vi "JKISM++ TopMain.vi"() -> ()   [LabVIEW 2014]
uses:
  user.lib/_NEVSTOP/JKI State Machine ++/_Support/JKISMQ/_JKISMQFGV.vi
  user.lib/_NEVSTOP/JKI State Machine ++/JKI-State-Machine-Plus.lvlib
panel:
  in  "List Module":bool
  out "Name":string[](array[string])
  in  "New Category: 3 -@A":bool
  in  "New Category: 3 ->A":bool
  in  "New Category: 2 -@B":bool
  out "State History":string
  in  "New Category: 2 ->B":bool
  in  "Boolean 1":bool
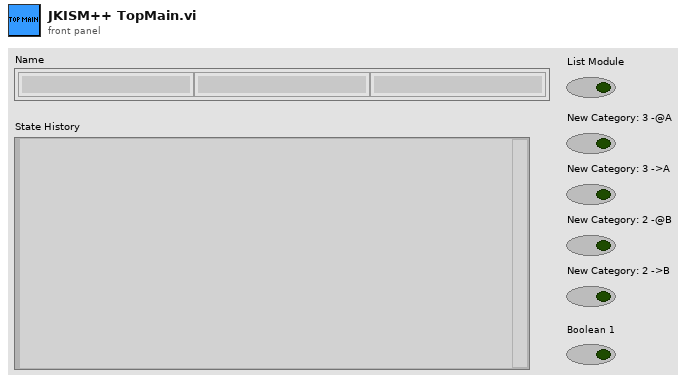
[diagram p1: front panel]
types:
  T1 = enum32{"Invalid", "Standard", "Closed", "Hidden", "Minimized", "Maximized"}
  T2 = enum32{"invalid app kind", "Development System", "Run Time System", "Student Edition", "Embedded LabVIEW", "Evaluation", "Custom"}
  T3 = cluster{"Core":cluster{"Current VI Reference":refnum<vi>, "Close Panel on Exit?":bool}, "Your Boolean data":bool, "Your string data":string}
  T4 = cluster{"Current VI Reference":refnum<vi>, "Close Panel on Exit?":bool}
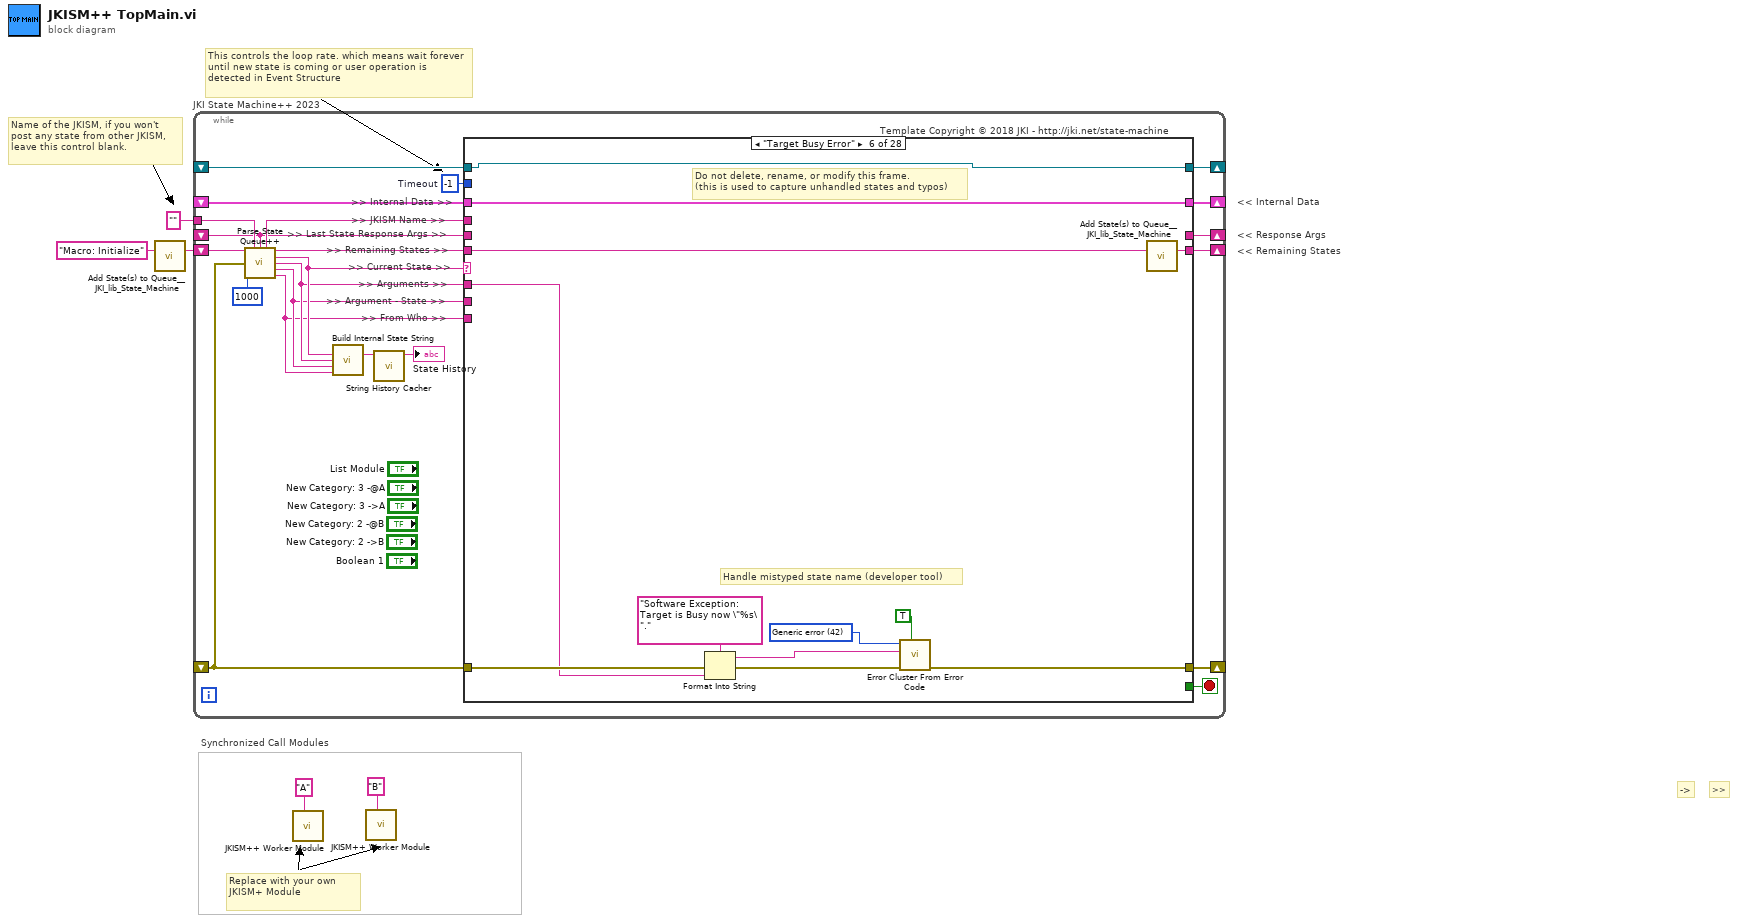
[diagram p0: block diagram]
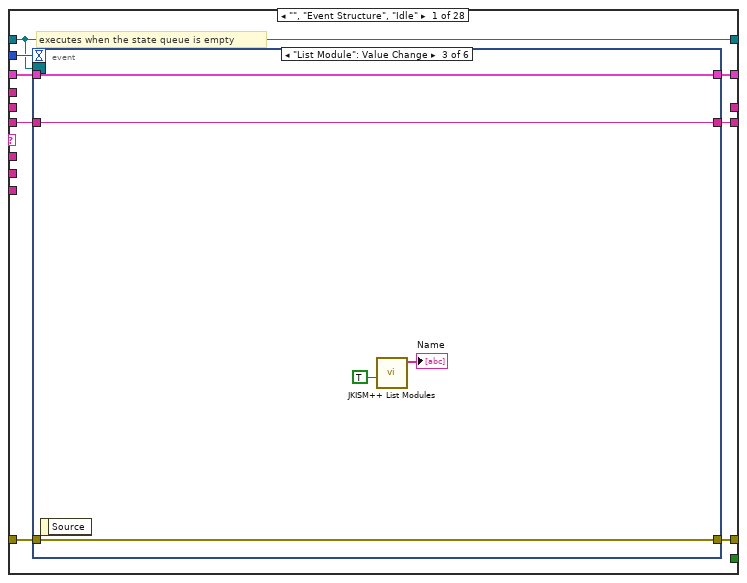
[diagram p2: hidden frame]
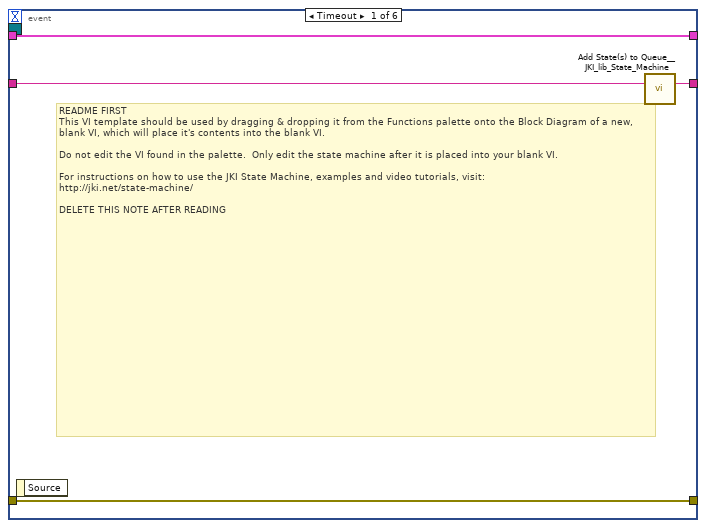
[diagram p3: hidden frame]
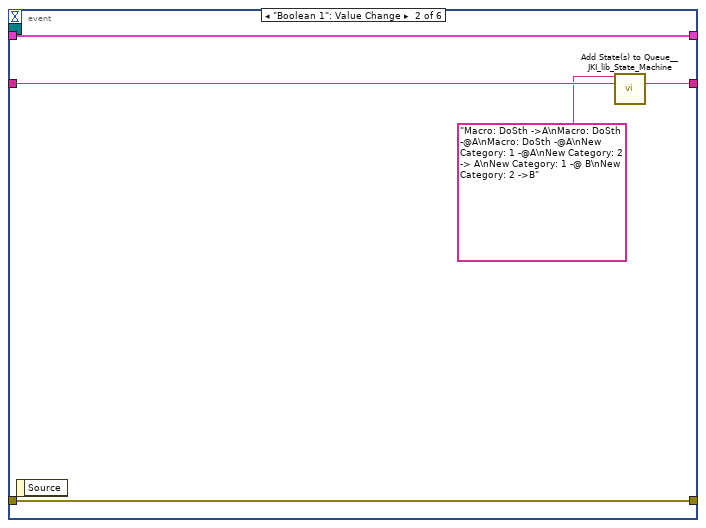
[diagram p4: hidden frame]
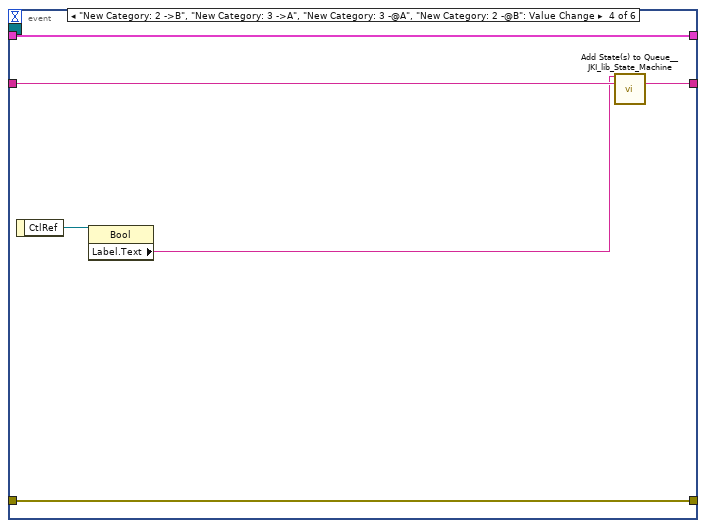
[diagram p5: hidden frame]
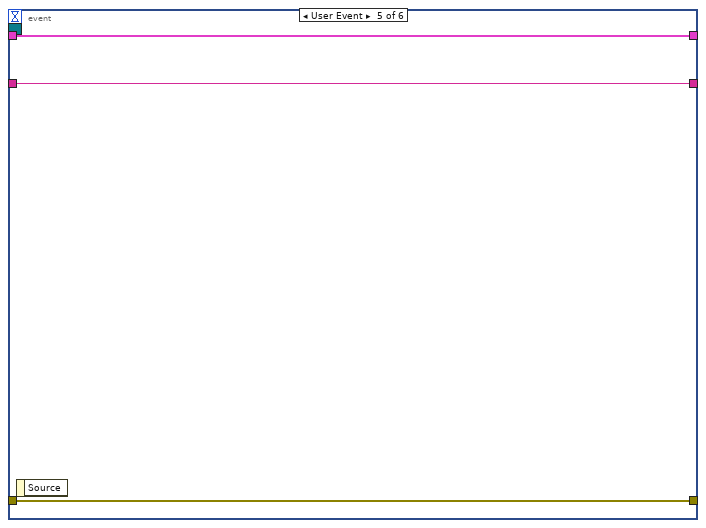
[diagram p6: hidden frame]
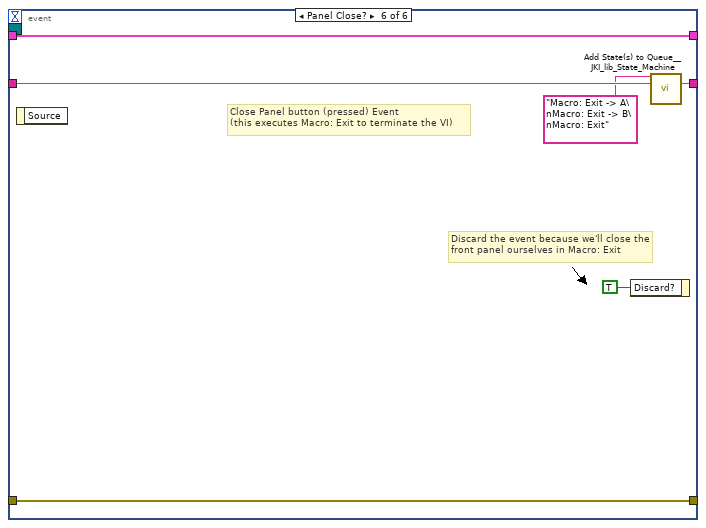
[diagram p7: hidden frame]
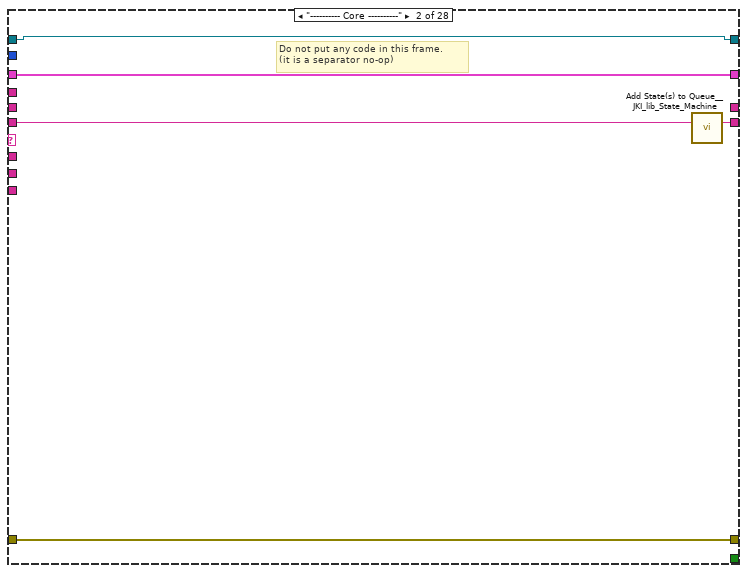
[diagram p8: hidden frame]
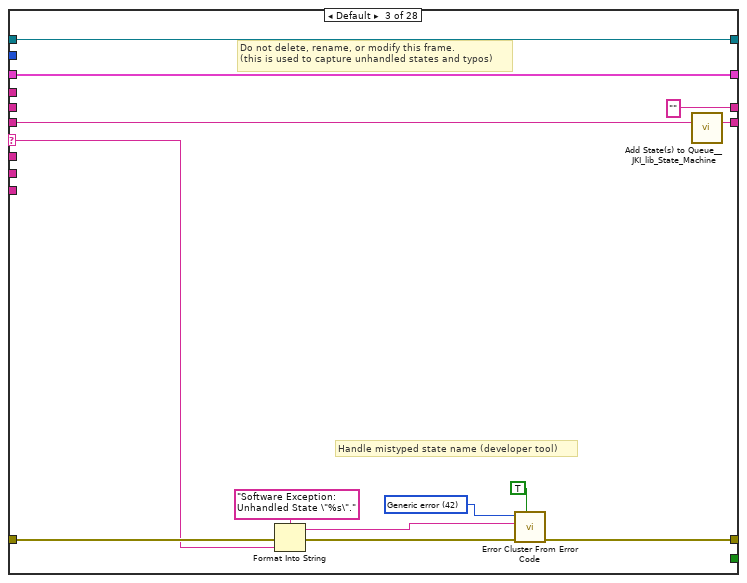
[diagram p9: hidden frame]
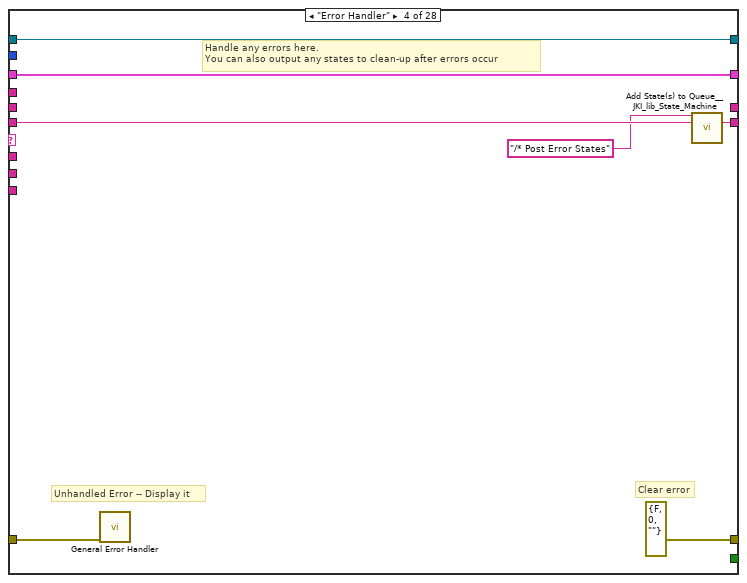
[diagram p10: hidden frame]
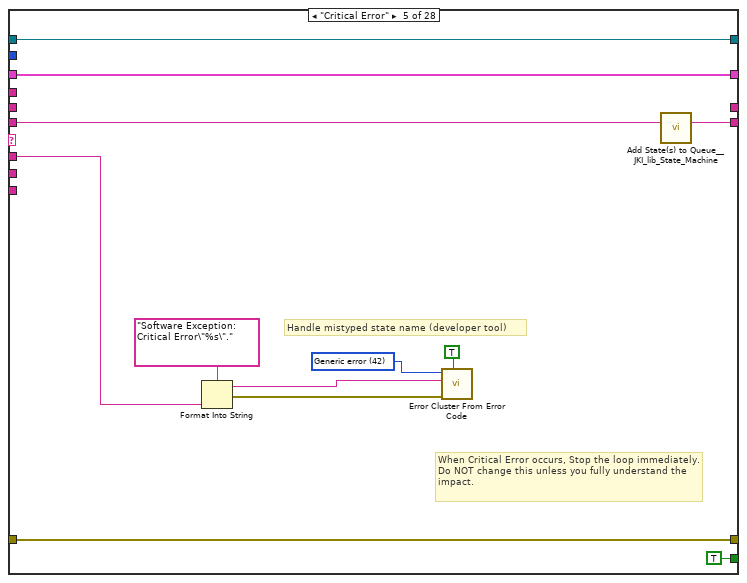
[diagram p11: hidden frame]
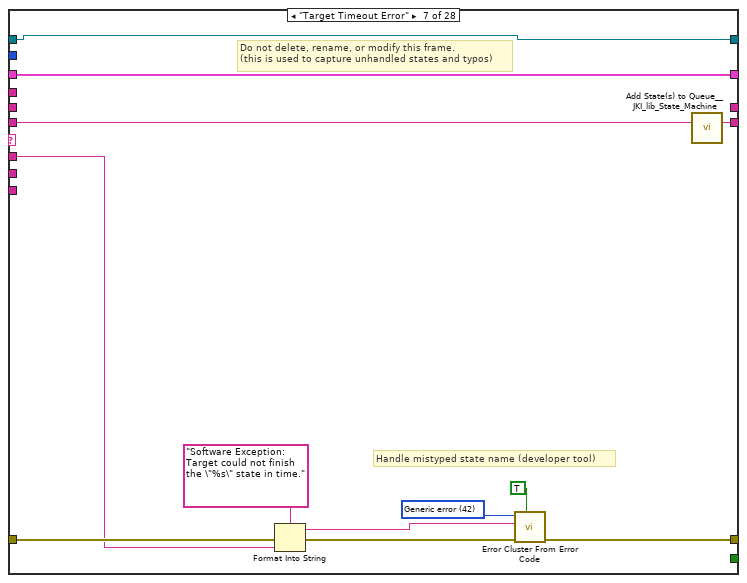
[diagram p12: hidden frame]
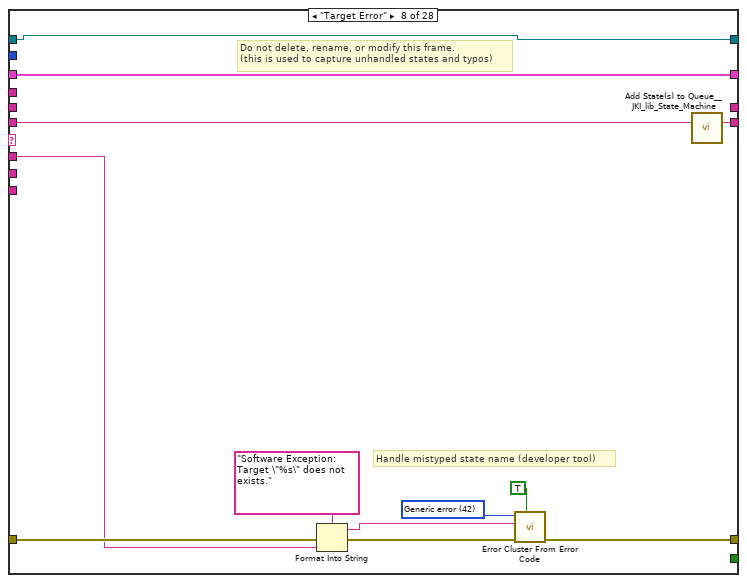
[diagram p13: hidden frame]
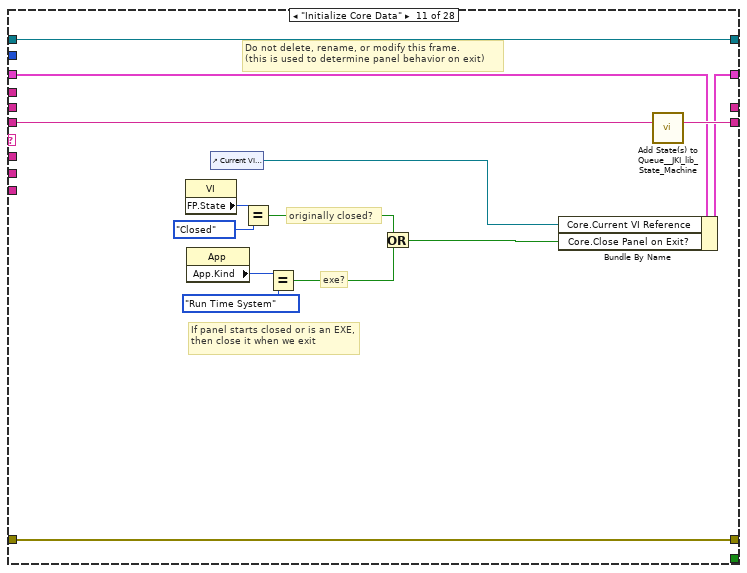
[diagram p16: hidden frame]
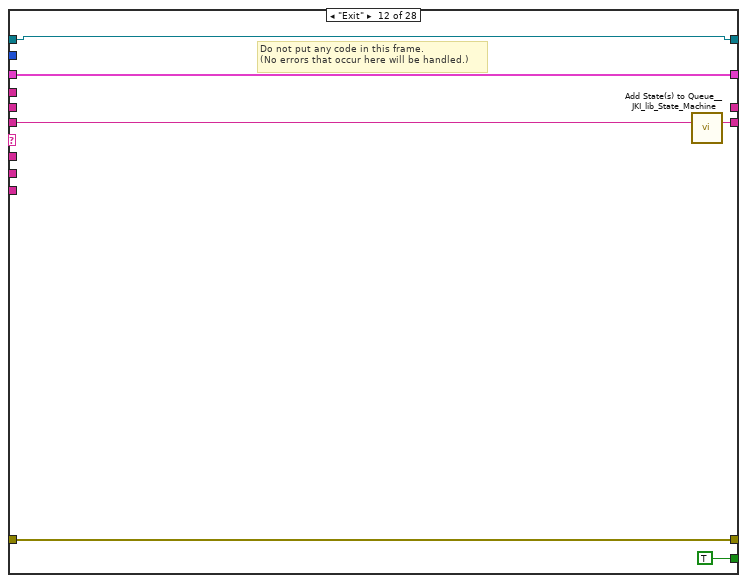
[diagram p17: hidden frame]
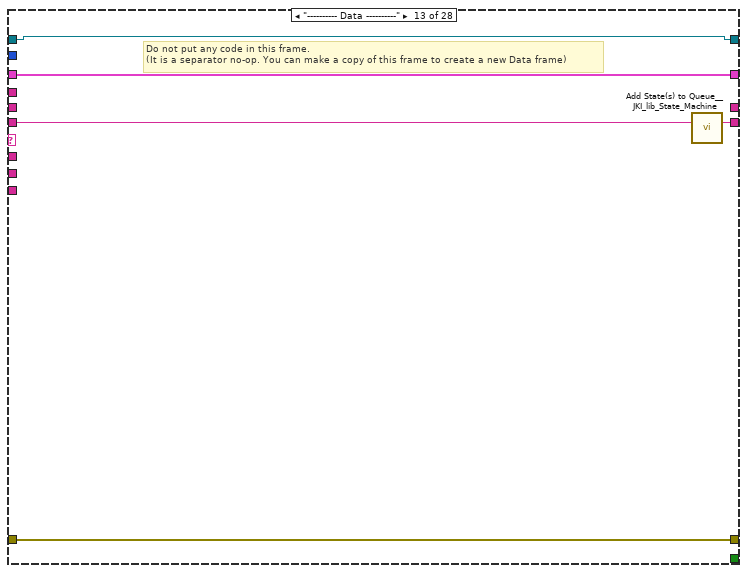
[diagram p18: hidden frame]
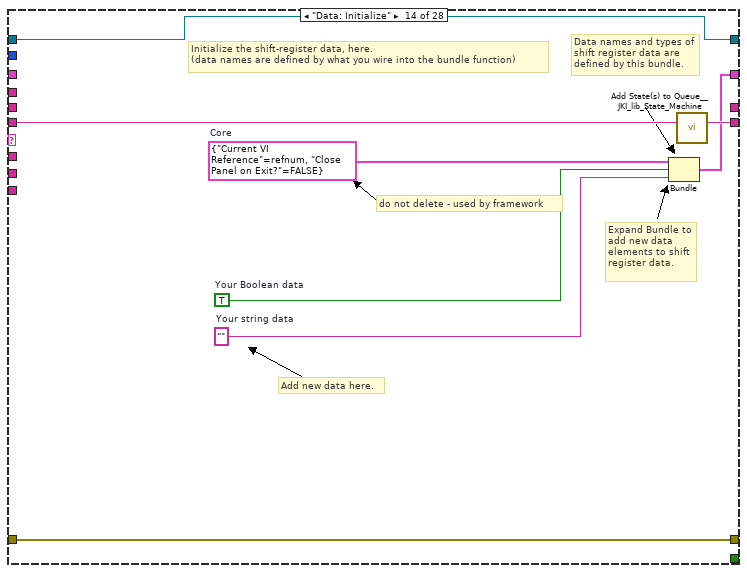
[diagram p19: hidden frame]
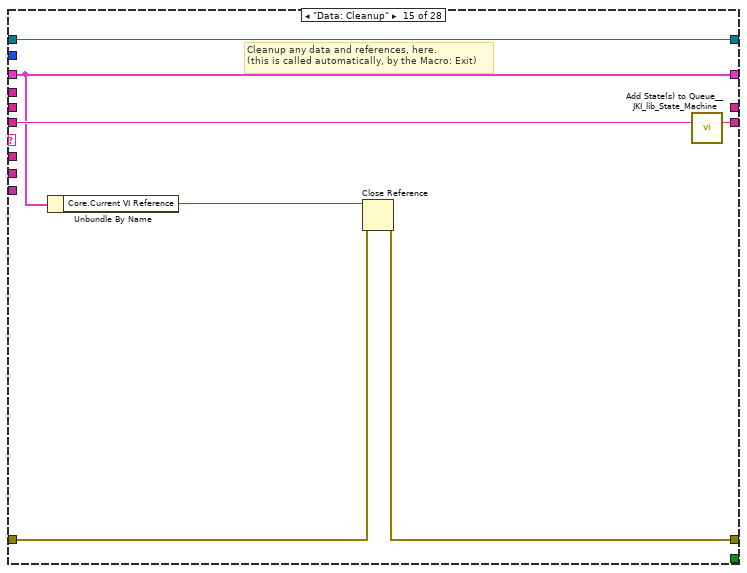
[diagram p20: hidden frame]
diagram:
  # ">>"
  # "->"
  # "<< Internal Data"
  # "<< Response Args"
  # "<< Remaining States"
  # "Name of the JKISM, if you won't post any state from other JKISM,  leave this control blank."
  # "This controls the loop rate. which means wait forever until new state is coming or user operation is detected in Event Structure"
  # "Synchronized Call Modules"
  # "Replace with your own JKISM+ Module"
  n1 = call <vilib>:"Add State(s) to Queue__JKI_lib_State_Machine.vi"("State(s) in (\"\")"="Macro: Initialize") -> ("States Out"=w3:string)  [unwired: 14 in]
  n2 = while "JKI State Machine++ 2023" {
    shift-right: [w22] -> _
    shift-left: _ -> [w21]
    shift-right: [w25] -> _
    shift-left: _ -> [w19]
    shift-right: [w24] -> _
    shift-left: w3 -> [w26]
    tunnel: "" ("Name(\"\" to use uuid)") -> [w14]
    shift-right: [w17] -> _
    shift-left: _ -> [w6]
    shift-right: [w16] -> _
    shift-left: _ -> [w15]
    stop <- w23 stop-if-true
    w20 = -1  # Timeout
    # ">> Internal Data >>"
    # ">> Last State Response Args >>"
    # ">> JKISM Name >>"
    # ">> From Who >>"
    # ">> Argument - State >>"
    # ">> Arguments >>"
    # ">> Current State >>"
    # ">> Remaining States >>"
    # "Template Copyright © 2018 JKI - http://jki.net/state-machine"
    n3 = call "Parse State Queue++.vi"("State Queue"=w26, "Name(\"\" to use uuid)"=w14, "Response Arguments"=w6, "Error In (no error)"=w19, "Response Timeout(5000ms)"=1000 ("Response Timeout(1000ms)")) -> ("Name Used"=w7:string, "Remaining States"=w27:string, "Current State"=w11:string, "Arguments"=w10:string, "Argument - State"=w9:string, "From Who"=w8:string)  [unwired: 5 in]
    n4 = call "Build Internal State String.vi"("State"=w11, "Arguments (\"\")"=w10, "Arg-State (\"\")"=w9, "Source (\"\")"=w8) -> ("State with Arguments"=w12:string)  [unwired: 11 in]
    n5 = call "String History Cacher.vi"("String"=w12) -> ("String Cache"=→"State History":string)  [unwired: 10 in]
    n6 = case shown="\"Target Busy Error\"" w11 {
      selector: w11 -> [_ _ w72 _ _ _ _ _ _ _ _ _ _ _ _ _ _ _ _ _ _ _ _ _ _ _ _ _]
      tunnel: w27 -> [w35 w69 w76 w89 w99 w107 w119 w131 w140 w144 w159 w165 w170 w178 w185 w190 w196 w200 w206 w211 w218 w230 w300 w306 w317 w322 w328 w334]
      tunnel: w10 -> [_ _ _ _ w92 w103 w115 w127 _ _ _ _ _ _ _ _ _ _ _ _ w213 w224 _ _ _ _ _ _]
      tunnel: w21 -> [w33 w66 w74 w86 w100 w105 w117 w129 w139 w143 w152 w163 w167 _ w180 w187 w195 w199 w203 w209 w216 w226 w297 w303 w314 w319 w325 w331]
      tunnel: [w32 w67 w78 errorcluster {"status"=FALSE, "code"=0, "source"=""} ("error out") w101 w109 w121 w133 w141 w145 w156 w162 w168 w175 w181 w188 w191 w198 w204 w208 w214 w227 w298 w304 w315 w320 w326 w332] -> w25
      tunnel: w19 -> [w31 w67 w77 w85 w101 w108 w120 w132 w141 w145 w156 w162 w168 w175 w182 w188 _ w201 w204 w208 w215 w228 w298 w304 w315 w320 w326 w332]
      tunnel: [w34 w68 w75 w88 w98 w106 w118 w130 w140 w144 w158 w164 w169 w177 w184 w189 w196 w200 w205 w210 w217 w229 w299 w305 w316 w321 w327 w333] -> w24
      tunnel: [_ _ _ _ TRUE _ _ _ _ _ _ TRUE _ _ _ _ _ _ _ _ _ _ _ _ _ _ _ _] -> w23
      tunnel: [w30 w66 w74 w86 w100 w105 w117 w129 w139 w143 w157 w163 w167 w176 w180 w187 w195 w199 w203 w209 w216 w226 w297 w303 w314 w319 w325 w331] -> w22
      tunnel: w20 -> [w29 _ _ _ _ _ _ _ _ _ _ _ _ _ _ _ _ _ _ _ _ _ _ _ _ _ _ _]
      tunnel: w8 -> [_ _ _ _ _ _ _ _ _ _ _ _ _ _ _ _ _ _ _ _ _ _ _ _ _ _ _ _]
      tunnel: w9 -> [_ _ _ _ _ _ _ _ _ _ _ _ _ _ _ _ _ _ _ _ _ _ _ _ _ _ _ _]
      tunnel: [_ _ "" _ _ _ _ _ _ _ _ _ _ _ _ _ _ _ _ _ _ _ _ _ _ _ "DoA Finished" "DoB Finished"] -> w17
      tunnel: [w28 w65 w70 w83 w90 w102 w114 w126 w138 w142 w146 w160 w166 w171 w179 w186 w194 w197 w202 w207 w212 w223 w296 w301 w307 w318 w324 w330] -> w16
      tunnel: w15 -> [w28 w65 w70 w83 w90 w102 w114 w126 w138 w142 w146 w160 w166 w171 w179 w186 _ w197 w202 w207 w212 w223 w296 w301 w307 w318 w324 w330]
      tunnel: w7 -> [_ _ _ _ _ _ _ _ _ _ _ _ _ _ _ _ w193 _ _ _ _ _ _ _ _ _ _ _]
      tunnel: w6 -> [_ _ _ _ _ _ _ _ _ _ _ _ _ _ _ _ _ _ _ _ _ _ _ _ _ _ _ _]
      frame "", "Event Structure", "Idle" {
        # "executes when the state queue is empty"
        n7 = event shown="[2] \"List Module\": Value Change" {
          selector: w28 -> [_ _ _ _ _ _]
          dyn-events: _ -> [_ _ _ _ _ _]
          timeout: w29 -> [_ _ _ _ _ _]
          tunnel: w35 -> [w39 w42 w49 w53 w57 w64]
          tunnel: [w38 w41 w49 w52 w57 w63] -> w34
          tunnel: w33 -> [w36 w43 w47 w54 w58 w61]
          tunnel: [w37 w44 w48 w55 w56 w62] -> w32
          tunnel: w31 -> [w37 w44 w48 w55 w56 w62]
          tunnel: [w36 w43 w47 w54 w58 w61] -> w30
          event Timeout {
            # "README FIRST\nThis VI template should be used by dragging & dropping it from the Functions palette onto the Block Diagram of a new, blank VI, which will place it's contents into the blank VI.\n\nDo not edit the VI found in the palette.  Only edit the state machine after it is placed into your blank VI.\n\nFor instructions on how to use the JKI State Machine, examples and video tutorials, visit:\nhttp://jki.net/state-machine/\n\nDELETE THIS NOTE AFTER READING"
            n8 = event-data() -> ()  [unwired: 1 in, 1 out]
            n9 = call <vilib>:"Add State(s) to Queue__JKI_lib_State_Machine.vi"("State(s) in (\"\")"=w39) -> ("States Out"=w38:string)  [unwired: 14 in]
          }
          event "Boolean 1": Value Change {
            n10 = event-data() -> ()  [unwired: 1 in, 1 out]
            n11 = call <vilib>:"Add State(s) to Queue__JKI_lib_State_Machine.vi"("State(s) in Front (\"\")"="Macro: DoSth ->A\nMacro: DoSth -@A\nMacro: DoSth -@A\nNew Category: 1 -@A\nNew Category: 2 -> A\nNew Category: 1 -@ B\nNew Category: 2 ->B" ("State(s) in Front (\"\")"), "State(s) in (\"\")"=w42) -> ("States Out"=w41:string)  [unwired: 13 in]
          }
          event "List Module": Value Change {
            n12 = event-data() -> ()  [unwired: 1 in, 1 out]
            n13 = call "JKISM++ List Modules.vi"("Exclude Standalone JKISM(T)"=TRUE) -> ("Name"=→"Name":string[])  [unwired: 9 in, 1 out]
          }
          event "New Category: 2 ->B", "New Category: 3 ->A", "New Category: 3 -@A", "New Category: 2 -@B": Value Change {
            n14 = event-data() -> ("CtlRef"=w51:refnum<vi>)  [unwired: 1 in]
            n15 = property class="Bool"(reference=w51) -> ("Label.Text"=w50:string)  [unwired: 1 in, 2 out]
            n16 = call <vilib>:"Add State(s) to Queue__JKI_lib_State_Machine.vi"("State(s) in Front (\"\")"=w50, "State(s) in (\"\")"=w53) -> ("States Out"=w52:string)  [unwired: 13 in]
          }
          event User Event {
            n17 = event-data() -> ()  [unwired: 1 in, 1 out]
          }
          event Panel Close? {
            # "Discard the event because we'll close the front panel ourselves in Macro: Exit"
            # "Close Panel button (pressed) Event\n(this executes Macro: Exit to terminate the VI)"
            n18 = event-data() -> ()  [unwired: 1 in, 1 out]
            n19 = event-data("Discard?"=TRUE) -> ()  [unwired: 1 in, 1 out]
            n20 = call <vilib>:"Add State(s) to Queue__JKI_lib_State_Machine.vi"("State(s) in Front (\"\")"="Macro: Exit -> A\nMacro: Exit -> B\nMacro: Exit", "State(s) in (\"\")"=w64) -> ("States Out"=w63:string)  [unwired: 13 in]
          }
        }
      }
      frame "---------- Core ----------" {
        # "Do not put any code in this frame.\n(it is a separator no-op)"
        n21 = call <vilib>:"Add State(s) to Queue__JKI_lib_State_Machine.vi"("State(s) in (\"\")"=w69) -> ("States Out"=w68:string)  [unwired: 14 in]
      }
      frame Default {
        w81 = 42 items=["No error", "Argument error", "Memory is full", "Out of zone", "End of file", "File already open", "Generic file I/O error", "File not found", "File permission error", "Disk is full", "Duplicate path", "Too many files open", "System feature not enabled", "Resource file not found", "Cannot add resource", "Resource not found", "Image not found", "Image memory error", "Pen does not exist", "Config type invalid", "Config token not found", "Config parse error", "Config memory error", "Bad external code format", "Bad external code offset", "External code not present", "Null window", "Destroy window error", "Null menu", "Print aborted", "Bad print record", "Print driver error", "Windows error during printing", "Memory error during printing", "Print dialog error", "Generic print error", "Invalid device refnum", "Device not found", "Device parameter error", "Device unit error", "Cannot open device", "Device call aborted", "Generic error", "Cancelled by user", "Object ID too low", "Object ID too high", "Object not in heap", "Unknown heap", "Unknown object (invalid DefProc)", "Unknown object (DefProc not in table)", "Message out of range", "Invalid (null) method", "Unknown message", "Manager call not supported", "Bad address", "Network operation in progress", "Network operation timed out", "Connection is busy", "Network attribute not supported", "Network error", "Address in use", "System out of memory", "Connection aborted", "Connection refused", "Not connected", "Already connected", "Connection closed", "Initialization error (interapplication manager)", "Bad occurrence", "Wait on unbound occurrence handler", "Occurrence queue overflow", "Datalog type conflict", "Unused", "Unrecognized type (interapplication manager)", "Memory corrupt", "Failed to make temporary DLL", "Old CIN version", "Drag socket not found", "Failed to load drop-object", "Failed to register OLE object", "Failed to release OLE object", "Format specifier type mismatch", "Unknown format specifier", "Too few format specifiers", "Too many format specifiers", "Scan failed", "Newer CIN version", "Error converting to variant", "Runtime menu error", "Password tampered", "Variant attribute not found", "Incompatible variant data type", "Event data is not available", "Event Store is not present", "Occurrence is not found", "Event Queue is not created", "Event info is not available", "Refnum passed is NULL", "Error retrieving Class GUID", "Error retrieving CoClass GUID", "Error retrieving TypeLib GUID.", "Bad built application magic bytes.", "Specific driver is different from the specific driver associated with the Logical Name.", "There is no session opened to the class driver.", "Max Error", "MAX - Error with config objects", "MAX - Error loading configuration", "MAX - Group not supported"]
        # "Do not delete, rename, or modify this frame.\n(this is used to capture unhandled states and typos)"
        # "Handle mistyped state name (developer tool)"
        n22 = Format Into String(format string="Software Exception: Unhandled State \"%s\"." ("message"), error in=w77, w72) -> (resulting string=w80:string, error out=w79:errorcluster)  [unwired: 1 in]
        n23 = call <vilib>:"Error Cluster From Error Code.vi"("show call chain? (False)"=TRUE, "error in (no error)"=w79, "error message (\"\")"=w80, "error code (0)"=w81) -> ("error out"=w78:errorcluster)  [unwired: 5 in]
        n24 = call <vilib>:"Add State(s) to Queue__JKI_lib_State_Machine.vi"("State(s) in (\"\")"=w76) -> ("States Out"=w75:string)  [unwired: 14 in]
      }
      frame "Error Handler" {
        # "Unhandled Error -- Display it"
        # "Handle any errors here.\nYou can also output any states to clean-up after errors occur"
        # "Clear error"
        n25 = call <vilib>:"General Error Handler.vi"("error in (no error)"=w85) -> ()  [unwired: 10 in, 5 out]
        n26 = call <vilib>:"Add State(s) to Queue__JKI_lib_State_Machine.vi"("State(s) in Front (\"\")"="/* Post Error States", "State(s) in (\"\")"=w89) -> ("States Out"=w88:string)  [unwired: 13 in]
      }
      frame "Critical Error" {
        w96 = 42 items=["No error", "Argument error", "Memory is full", "Out of zone", "End of file", "File already open", "Generic file I/O error", "File not found", "File permission error", "Disk is full", "Duplicate path", "Too many files open", "System feature not enabled", "Resource file not found", "Cannot add resource", "Resource not found", "Image not found", "Image memory error", "Pen does not exist", "Config type invalid", "Config token not found", "Config parse error", "Config memory error", "Bad external code format", "Bad external code offset", "External code not present", "Null window", "Destroy window error", "Null menu", "Print aborted", "Bad print record", "Print driver error", "Windows error during printing", "Memory error during printing", "Print dialog error", "Generic print error", "Invalid device refnum", "Device not found", "Device parameter error", "Device unit error", "Cannot open device", "Device call aborted", "Generic error", "Cancelled by user", "Object ID too low", "Object ID too high", "Object not in heap", "Unknown heap", "Unknown object (invalid DefProc)", "Unknown object (DefProc not in table)", "Message out of range", "Invalid (null) method", "Unknown message", "Manager call not supported", "Bad address", "Network operation in progress", "Network operation timed out", "Connection is busy", "Network attribute not supported", "Network error", "Address in use", "System out of memory", "Connection aborted", "Connection refused", "Not connected", "Already connected", "Connection closed", "Initialization error (interapplication manager)", "Bad occurrence", "Wait on unbound occurrence handler", "Occurrence queue overflow", "Datalog type conflict", "Unused", "Unrecognized type (interapplication manager)", "Memory corrupt", "Failed to make temporary DLL", "Old CIN version", "Drag socket not found", "Failed to load drop-object", "Failed to register OLE object", "Failed to release OLE object", "Format specifier type mismatch", "Unknown format specifier", "Too few format specifiers", "Too many format specifiers", "Scan failed", "Newer CIN version", "Error converting to variant", "Runtime menu error", "Password tampered", "Variant attribute not found", "Incompatible variant data type", "Event data is not available", "Event Store is not present", "Occurrence is not found", "Event Queue is not created", "Event info is not available", "Refnum passed is NULL", "Error retrieving Class GUID", "Error retrieving CoClass GUID", "Error retrieving TypeLib GUID.", "Bad built application magic bytes.", "Specific driver is different from the specific driver associated with the Logical Name.", "There is no session opened to the class driver.", "Max Error", "MAX - Error with config objects", "MAX - Error loading configuration", "MAX - Group not supported"]
        # "When Critical Error occurs, Stop the loop immediately. Do NOT change this unless you fully understand the impact."
        # "Handle mistyped state name (developer tool)"
        n27 = Format Into String(format string="Software Exception: Critical Error\"%s\"." ("message"), w92) -> (resulting string=w95:string, error out=w94:errorcluster)  [unwired: 2 in]
        n28 = call <vilib>:"Error Cluster From Error Code.vi"("show call chain? (False)"=TRUE, "error in (no error)"=w94, "error message (\"\")"=w95, "error code (0)"=w96) -> ()  [unwired: 5 in, 1 out]
        n29 = call <vilib>:"Add State(s) to Queue__JKI_lib_State_Machine.vi"("State(s) in (\"\")"=w99) -> ("States Out"=w98:string)  [unwired: 14 in]
      }
      frame "Target Busy Error" {
        w112 = 42 items=["No error", "Argument error", "Memory is full", "Out of zone", "End of file", "File already open", "Generic file I/O error", "File not found", "File permission error", "Disk is full", "Duplicate path", "Too many files open", "System feature not enabled", "Resource file not found", "Cannot add resource", "Resource not found", "Image not found", "Image memory error", "Pen does not exist", "Config type invalid", "Config token not found", "Config parse error", "Config memory error", "Bad external code format", "Bad external code offset", "External code not present", "Null window", "Destroy window error", "Null menu", "Print aborted", "Bad print record", "Print driver error", "Windows error during printing", "Memory error during printing", "Print dialog error", "Generic print error", "Invalid device refnum", "Device not found", "Device parameter error", "Device unit error", "Cannot open device", "Device call aborted", "Generic error", "Cancelled by user", "Object ID too low", "Object ID too high", "Object not in heap", "Unknown heap", "Unknown object (invalid DefProc)", "Unknown object (DefProc not in table)", "Message out of range", "Invalid (null) method", "Unknown message", "Manager call not supported", "Bad address", "Network operation in progress", "Network operation timed out", "Connection is busy", "Network attribute not supported", "Network error", "Address in use", "System out of memory", "Connection aborted", "Connection refused", "Not connected", "Already connected", "Connection closed", "Initialization error (interapplication manager)", "Bad occurrence", "Wait on unbound occurrence handler", "Occurrence queue overflow", "Datalog type conflict", "Unused", "Unrecognized type (interapplication manager)", "Memory corrupt", "Failed to make temporary DLL", "Old CIN version", "Drag socket not found", "Failed to load drop-object", "Failed to register OLE object", "Failed to release OLE object", "Format specifier type mismatch", "Unknown format specifier", "Too few format specifiers", "Too many format specifiers", "Scan failed", "Newer CIN version", "Error converting to variant", "Runtime menu error", "Password tampered", "Variant attribute not found", "Incompatible variant data type", "Event data is not available", "Event Store is not present", "Occurrence is not found", "Event Queue is not created", "Event info is not available", "Refnum passed is NULL", "Error retrieving Class GUID", "Error retrieving CoClass GUID", "Error retrieving TypeLib GUID.", "Bad built application magic bytes.", "Specific driver is different from the specific driver associated with the Logical Name.", "There is no session opened to the class driver.", "Max Error", "MAX - Error with config objects", "MAX - Error loading configuration", "MAX - Group not supported"]
        # "Do not delete, rename, or modify this frame.\n(this is used to capture unhandled states and typos)"
        # "Handle mistyped state name (developer tool)"
        n30 = Format Into String(format string="Software Exception: Target is Busy now \"%s\"." ("message"), error in=w108, w103) -> (resulting string=w111:string, error out=w110:errorcluster)  [unwired: 1 in]
        n31 = call <vilib>:"Error Cluster From Error Code.vi"("show call chain? (False)"=TRUE, "error in (no error)"=w110, "error message (\"\")"=w111, "error code (0)"=w112) -> ("error out"=w109:errorcluster)  [unwired: 5 in]
        n32 = call <vilib>:"Add State(s) to Queue__JKI_lib_State_Machine.vi"("State(s) in (\"\")"=w107) -> ("States Out"=w106:string)  [unwired: 14 in]
      }
      frame "Target Timeout Error" {
        w124 = 42 items=["No error", "Argument error", "Memory is full", "Out of zone", "End of file", "File already open", "Generic file I/O error", "File not found", "File permission error", "Disk is full", "Duplicate path", "Too many files open", "System feature not enabled", "Resource file not found", "Cannot add resource", "Resource not found", "Image not found", "Image memory error", "Pen does not exist", "Config type invalid", "Config token not found", "Config parse error", "Config memory error", "Bad external code format", "Bad external code offset", "External code not present", "Null window", "Destroy window error", "Null menu", "Print aborted", "Bad print record", "Print driver error", "Windows error during printing", "Memory error during printing", "Print dialog error", "Generic print error", "Invalid device refnum", "Device not found", "Device parameter error", "Device unit error", "Cannot open device", "Device call aborted", "Generic error", "Cancelled by user", "Object ID too low", "Object ID too high", "Object not in heap", "Unknown heap", "Unknown object (invalid DefProc)", "Unknown object (DefProc not in table)", "Message out of range", "Invalid (null) method", "Unknown message", "Manager call not supported", "Bad address", "Network operation in progress", "Network operation timed out", "Connection is busy", "Network attribute not supported", "Network error", "Address in use", "System out of memory", "Connection aborted", "Connection refused", "Not connected", "Already connected", "Connection closed", "Initialization error (interapplication manager)", "Bad occurrence", "Wait on unbound occurrence handler", "Occurrence queue overflow", "Datalog type conflict", "Unused", "Unrecognized type (interapplication manager)", "Memory corrupt", "Failed to make temporary DLL", "Old CIN version", "Drag socket not found", "Failed to load drop-object", "Failed to register OLE object", "Failed to release OLE object", "Format specifier type mismatch", "Unknown format specifier", "Too few format specifiers", "Too many format specifiers", "Scan failed", "Newer CIN version", "Error converting to variant", "Runtime menu error", "Password tampered", "Variant attribute not found", "Incompatible variant data type", "Event data is not available", "Event Store is not present", "Occurrence is not found", "Event Queue is not created", "Event info is not available", "Refnum passed is NULL", "Error retrieving Class GUID", "Error retrieving CoClass GUID", "Error retrieving TypeLib GUID.", "Bad built application magic bytes.", "Specific driver is different from the specific driver associated with the Logical Name.", "There is no session opened to the class driver.", "Max Error", "MAX - Error with config objects", "MAX - Error loading configuration", "MAX - Group not supported"]
        # "Do not delete, rename, or modify this frame.\n(this is used to capture unhandled states and typos)"
        # "Handle mistyped state name (developer tool)"
        n33 = Format Into String(format string="Software Exception: Target could not finish the \"%s\" state in time." ("message"), error in=w120, w115) -> (resulting string=w123:string, error out=w122:errorcluster)  [unwired: 1 in]
        n34 = call <vilib>:"Error Cluster From Error Code.vi"("show call chain? (False)"=TRUE, "error in (no error)"=w122, "error message (\"\")"=w123, "error code (0)"=w124) -> ("error out"=w121:errorcluster)  [unwired: 5 in]
        n35 = call <vilib>:"Add State(s) to Queue__JKI_lib_State_Machine.vi"("State(s) in (\"\")"=w119) -> ("States Out"=w118:string)  [unwired: 14 in]
      }
      frame "Target Error" {
        w136 = 42 items=["No error", "Argument error", "Memory is full", "Out of zone", "End of file", "File already open", "Generic file I/O error", "File not found", "File permission error", "Disk is full", "Duplicate path", "Too many files open", "System feature not enabled", "Resource file not found", "Cannot add resource", "Resource not found", "Image not found", "Image memory error", "Pen does not exist", "Config type invalid", "Config token not found", "Config parse error", "Config memory error", "Bad external code format", "Bad external code offset", "External code not present", "Null window", "Destroy window error", "Null menu", "Print aborted", "Bad print record", "Print driver error", "Windows error during printing", "Memory error during printing", "Print dialog error", "Generic print error", "Invalid device refnum", "Device not found", "Device parameter error", "Device unit error", "Cannot open device", "Device call aborted", "Generic error", "Cancelled by user", "Object ID too low", "Object ID too high", "Object not in heap", "Unknown heap", "Unknown object (invalid DefProc)", "Unknown object (DefProc not in table)", "Message out of range", "Invalid (null) method", "Unknown message", "Manager call not supported", "Bad address", "Network operation in progress", "Network operation timed out", "Connection is busy", "Network attribute not supported", "Network error", "Address in use", "System out of memory", "Connection aborted", "Connection refused", "Not connected", "Already connected", "Connection closed", "Initialization error (interapplication manager)", "Bad occurrence", "Wait on unbound occurrence handler", "Occurrence queue overflow", "Datalog type conflict", "Unused", "Unrecognized type (interapplication manager)", "Memory corrupt", "Failed to make temporary DLL", "Old CIN version", "Drag socket not found", "Failed to load drop-object", "Failed to register OLE object", "Failed to release OLE object", "Format specifier type mismatch", "Unknown format specifier", "Too few format specifiers", "Too many format specifiers", "Scan failed", "Newer CIN version", "Error converting to variant", "Runtime menu error", "Password tampered", "Variant attribute not found", "Incompatible variant data type", "Event data is not available", "Event Store is not present", "Occurrence is not found", "Event Queue is not created", "Event info is not available", "Refnum passed is NULL", "Error retrieving Class GUID", "Error retrieving CoClass GUID", "Error retrieving TypeLib GUID.", "Bad built application magic bytes.", "Specific driver is different from the specific driver associated with the Logical Name.", "There is no session opened to the class driver.", "Max Error", "MAX - Error with config objects", "MAX - Error loading configuration", "MAX - Group not supported"]
        # "Do not delete, rename, or modify this frame.\n(this is used to capture unhandled states and typos)"
        # "Handle mistyped state name (developer tool)"
        n36 = Format Into String(format string="Software Exception: Target \"%s\" does not exists." ("message"), error in=w132, w127) -> (resulting string=w135:string, error out=w134:errorcluster)  [unwired: 1 in]
        n37 = call <vilib>:"Error Cluster From Error Code.vi"("show call chain? (False)"=TRUE, "error in (no error)"=w134, "error message (\"\")"=w135, "error code (0)"=w136) -> ("error out"=w133:errorcluster)  [unwired: 5 in]
        n38 = call <vilib>:"Add State(s) to Queue__JKI_lib_State_Machine.vi"("State(s) in (\"\")"=w131) -> ("States Out"=w130:string)  [unwired: 14 in]
      }
      frame "Async Response", "Response" {
      }
      frame "Async Message Posted" {
      }
      frame "Initialize Core Data" {
        # "Do not delete, rename, or modify this frame.\n(this is used to determine panel behavior on exit)"
        # "originally closed?"
        # "exe?"
        # "If panel starts closed or is an EXE, then close it when we exit"
        n39 = property class="VI"() -> ("FP.State"=w149:T1)  [unwired: 2 in, 2 out]
        n40 = property class="App"() -> ("App.Kind"=w155:T2)  [unwired: 2 in, 2 out]
        n41 = control-ref of="Current VI Reference"() -> (w150:refnum<vi>)
        n42 = Equal?(x=w149, y=T1."Closed" ("Front Panel Window:State")) -> (x = y?=w147:bool)
        n43 = Equal?(x=w155, y=T2."Run Time System" ("Application:Kind")) -> (x = y?=w153:bool)
        n44 = Or(x=w147, y=w153) -> (x .or. y?=w151:bool)
        n45 = Bundle By Name(cluster=w152, "Core.Current VI Reference"=w150, "Core.Close Panel on Exit?"=w151) -> (w157:T3)
        n46 = call <vilib>:"Add State(s) to Queue__JKI_lib_State_Machine.vi"("State(s) in (\"\")"=w159) -> ("States Out"=w158:string)  [unwired: 14 in]
      }
      frame "Exit" {
        # "Do not put any code in this frame.\n(No errors that occur here will be handled.)"
        n47 = call <vilib>:"Add State(s) to Queue__JKI_lib_State_Machine.vi"("State(s) in (\"\")"=w165) -> ("States Out"=w164:string)  [unwired: 14 in]
      }
      frame "---------- Data ----------" {
        # "Do not put any code in this frame.\n(It is a separator no-op. You can make a copy of this frame to create a new Data frame)"
        n48 = call <vilib>:"Add State(s) to Queue__JKI_lib_State_Machine.vi"("State(s) in (\"\")"=w170) -> ("States Out"=w169:string)  [unwired: 14 in]
      }
      frame "Data: Initialize" {
        w172 = T4 {"Current VI Reference"=refnum, "Close Panel on Exit?"=FALSE}  # Core
        w174 = TRUE  # Your Boolean data
        w173 = ""  # Your string data
        # "do not delete - used by framework"
        # "Expand Bundle to add new data elements to shift register data."
        # "Add new data here."
        # "Data names and types of shift register data are defined by this bundle."
        # "Initialize the shift-register data, here.\n(data names are defined by what you wire into the bundle function)"
        n49 = Bundle("Core"=w172, "Your Boolean data"=w174, "Your string data"=w173) -> (w176:T3)  [unwired: 1 in]
        n50 = call <vilib>:"Add State(s) to Queue__JKI_lib_State_Machine.vi"("State(s) in (\"\")"=w178) -> ("States Out"=w177:string)  [unwired: 14 in]
      }
      frame "Data: Cleanup" {
        # "Cleanup any data and references, here.\n(this is called automatically, by the Macro: Exit)"
        n51 = Unbundle By Name(w180) -> ("Core.Current VI Reference"=w183:refnum<vi>)
        n52 = Close Reference(reference=w183, error in (no error)=w182) -> (error out=w181:errorcluster)
        n53 = call <vilib>:"Add State(s) to Queue__JKI_lib_State_Machine.vi"("State(s) in (\"\")"=w185) -> ("States Out"=w184:string)  [unwired: 14 in]
      }
      frame "---------- Events ----------" {
        # "Do not put any code in this frame.\n(It is a separator no-op. You can make a copy of this frame to create a new UI frame)"
        n54 = call <vilib>:"Add State(s) to Queue__JKI_lib_State_Machine.vi"("State(s) in (\"\")"=w190) -> ("States Out"=w189:string)  [unwired: 14 in]
      }
      frame "Events: Register" {
        n55 = call "JKISM++ Get New State Notifier Event.vi"("Name(\"\" to use uuid) in"=w193) -> ("Error out"=w191:errorcluster, "New State Notifier Event"=w192:refnum<user-event>)  [unwired: 9 in]
        n56 = register-events(w192) -> (reference out=w194:refnum<event-registration>)  [unwired: 2 in, 1 out]
      }
      frame "Events: Unregister" {
        n57 = Unregister For Events(event registration refnum=w197, error in=w201) -> (error out=w198:errorcluster)
      }
      frame "---------- UI ----------" {
        # "Do not put any code in this frame.\n(It is a separator no-op. You can make a copy of this frame to create a new UI frame)"
        n58 = call <vilib>:"Add State(s) to Queue__JKI_lib_State_Machine.vi"("State(s) in (\"\")"=w206) -> ("States Out"=w205:string)  [unwired: 14 in]
      }
      frame "UI: Initialize" {
        # "Initialize the User Interface, here.\n(this is called automatically, by the Macro: Init)"
        n59 = call <vilib>:"Add State(s) to Queue__JKI_lib_State_Machine.vi"("State(s) in (\"\")"=w211) -> ("States Out"=w210:string)  [unwired: 14 in]
      }
      frame "UI: Cursor Set" {
        # "Argument"
        # "Set and Unset Cursor Busy.\n(Usage: \"UI: Cursor Set >> Busy|Idle\")"
        n60 = case shown="\"Idle\", Default" w213 {
          tunnel: w215 -> [w220 w222]
          tunnel: [w219 w221] -> w214
          frame "Idle", Default {
            n61 = call <vilib>:"Unset Busy.vi"("error in (no error)"=w220) -> ("error out"=w219:errorcluster)  [unwired: 10 in]
          }
          frame "Busy" {
            n62 = call <vilib>:"Set Busy.vi"("error in (no error)"=w222) -> ("error out"=w221:errorcluster)  [unwired: 9 in, 1 out]
          }
        }
        n63 = call <vilib>:"Add State(s) to Queue__JKI_lib_State_Machine.vi"("State(s) in (\"\")"=w218) -> ("States Out"=w217:string)  [unwired: 14 in]
      }
      frame "UI: Front Panel State" {
        # "Argument"
        # "Set Front Panel Open or Closed\n(Usage: \"UI: Front Panel State >> Open|Close\")"
        n64 = Unbundle By Name(w226) -> ("Core.Current VI Reference"=w225:refnum<vi>)
        n65 = case shown="\"Minimize\", \"Minimized\"" w224 {
          tunnel: w228 -> [w236 w251 w262 w275 w288]
          tunnel: [w238 w252 w264 w277 w290] -> w227
          tunnel: w225 -> [w237 w249 w263 w276 w289]
          frame "Open", "Standard", Default {
            w231 = T1."Standard" ("State")
            n66 = property class="VI"(reference=w237, error in=w236) -> (reference out=w234:refnum<vi>, error out=w235:errorcluster, "FP.State"=w233:T1)
            n67 = Not Equal?(x=w233, y=w231) -> (x != y?=w232:bool)
            n68 = case shown="True" w232 {
              tunnel: [w242 w244] -> w238
              tunnel: w235 -> [w241 w244]
              tunnel: w234 -> [w240 _]
              tunnel: w231 -> [w239 _]
              frame True {
                n69 = invoke class="VI" method="FP.Open"(reference=w240, error in=w241, "Activate"=TRUE, "State"=w239) -> (error out=w242:errorcluster)  [unwired: 1 in, 4 out]
              }
              frame False {
              }
            }
          }
          frame "Close", "Closed" {
            n70 = property class="VI"(reference=w249, error in=w251) -> (reference out=w248:refnum<vi>, error out=w250:errorcluster, "FP.State"=w246:T1)
            n71 = Not Equal?(x=w246, y=T1."Closed" ("Front Panel Window:State")) -> (x != y?=w245:bool)
            n72 = case shown="True" w245 {
              tunnel: [w253 w256] -> w252
              tunnel: w250 -> [w253 w255]
              tunnel: w248 -> [_ w254]
              frame False {
              }
              frame True {
                n73 = invoke class="VI" method="FP.Close"(reference=w254, error in=w255) -> (error out=w256:errorcluster)  [unwired: 1 in, 2 out]
              }
            }
          }
          frame "Hidden", "Hide" {
            w257 = T1."Hidden" ("State")
            n74 = property class="VI"(reference=w263, error in=w262) -> (reference out=w260:refnum<vi>, error out=w261:errorcluster, "FP.State"=w259:T1)
            n75 = Not Equal?(x=w259, y=w257) -> (x != y?=w258:bool)
            n76 = case shown="True" w258 {
              tunnel: [w268 w269] -> w264
              tunnel: w261 -> [w267 w269]
              tunnel: w260 -> [w266 _]
              tunnel: w257 -> [w265 _]
              frame True {
                n77 = invoke class="VI" method="FP.Open"(reference=w266, error in=w267, "State"=w265) -> (error out=w268:errorcluster)  [unwired: 2 in, 4 out]
              }
              frame False {
              }
            }
          }
          frame "Minimize", "Minimized" {
            w270 = T1."Minimized" ("State")
            n78 = property class="VI"(reference=w276, error in=w275) -> (reference out=w273:refnum<vi>, error out=w274:errorcluster, "FP.State"=w272:T1)
            n79 = Not Equal?(x=w272, y=w270) -> (x != y?=w271:bool)
            n80 = case shown="True" w271 {
              tunnel: [w281 w282] -> w277
              tunnel: w274 -> [w280 w282]
              tunnel: w273 -> [w279 _]
              tunnel: w270 -> [w278 _]
              frame True {
                n81 = invoke class="VI" method="FP.Open"(reference=w279, error in=w280, "State"=w278) -> (error out=w281:errorcluster)  [unwired: 2 in, 4 out]
              }
              frame False {
              }
            }
          }
          frame "Maximize", "Maximized" {
            w283 = T1."Maximized" ("State")
            n82 = property class="VI"(reference=w289, error in=w288) -> (reference out=w286:refnum<vi>, error out=w287:errorcluster, "FP.State"=w285:T1)
            n83 = Not Equal?(x=w285, y=w283) -> (x != y?=w284:bool)
            n84 = case shown="True" w284 {
              tunnel: [w294 w295] -> w290
              tunnel: w287 -> [w293 w295]
              tunnel: w286 -> [w292 _]
              tunnel: w283 -> [w291 _]
              frame True {
                n85 = invoke class="VI" method="FP.Open"(reference=w292, error in=w293, "State"=w291) -> (error out=w294:errorcluster)  [unwired: 2 in, 4 out]
              }
              frame False {
              }
            }
          }
        }
        n86 = call <vilib>:"Add State(s) to Queue__JKI_lib_State_Machine.vi"("State(s) in (\"\")"=w230) -> ("States Out"=w229:string)  [unwired: 14 in]
      }
      frame "---------- Macro ----------" {
        # "Do not put any code in this frame.\n(It is a separator no-op. You can make a copy of this frame to create a new Macro frame)"
        n87 = call <vilib>:"Add State(s) to Queue__JKI_lib_State_Machine.vi"("State(s) in (\"\")"=w300) -> ("States Out"=w299:string)  [unwired: 14 in]
      }
      frame "Macro: Initialize" {
        w302 = "Data: Initialize\nInitialize Core Data\nEvents: Register\nUI: Initialize\nUI: Front Panel State >> Open"  # Data: Initialize Initialize Core Data Events: Register UI: Initialize UI: Front Panel State >> Open
        # "Initialization Macro\n(This is called once, when the VI starts)"
        n88 = call <vilib>:"Add State(s) to Queue__JKI_lib_State_Machine.vi"("State(s) in Front (\"\")"=w302, "State(s) in (\"\")"=w306) -> ("States Out"=w305:string)  [unwired: 13 in]
      }
      frame "Macro: Exit" {
        # "Exit Macro\n(This is called once, when the VI exits)"
        n89 = Unbundle By Name(w314) -> ("Core.Close Panel on Exit?"=w313:bool)
        n90 = Select(t="UI: Front Panel State >> Close", s=w313, f="") -> (s? t:f=w310:string)
        n91 = call <vilib>:"Add State(s) to Queue__JKI_lib_State_Machine.vi"("State(s) in (\"\")"=w310, "State(s) at Back (\"\")"="Data: Cleanup\nEvents: Unregister\nExit") -> ("States Out"=w308:string)  [unwired: 13 in]
        n92 = call <vilib>:"Add State(s) to Queue__JKI_lib_State_Machine.vi"("State(s) in Front (\"\")"=w308, "State(s) in (\"\")"=w317) -> ("States Out"=w316:string)  [unwired: 13 in]
      }
      frame "---------- DoSth ----------" {
        # "Template Separator\n(You can make a copy of, or modify, this frame)"
        n93 = call <vilib>:"Add State(s) to Queue__JKI_lib_State_Machine.vi"("State(s) in (\"\")"=w322) -> ("States Out"=w321:string)  [unwired: 14 in]
      }
      frame "DoSth: DoA" {
        # "Your code here.\n(You can make a copy of, or modify, this frame)"
        n94 = call <vilib>:"Add State(s) to Queue__JKI_lib_State_Machine.vi"("State(s) in (\"\")"=w328) -> ("States Out"=w327:string)  [unwired: 14 in]
      }
      frame "DoSth: DoB" {
        # "Your code here.\n(You can make a copy of, or modify, this frame)"
        n95 = call <vilib>:"Add State(s) to Queue__JKI_lib_State_Machine.vi"("State(s) in (\"\")"=w334) -> ("States Out"=w333:string)  [unwired: 14 in]
      }
    }
  }
  n96 = call "JKISM++ Worker Module.vi"("Name(\"\" to use uuid)"="A" ("Name")) -> ()  [unwired: 11 in]
  n97 = call "JKISM++ Worker Module.vi"("Name(\"\" to use uuid)"="B" ("Name")) -> ()  [unwired: 11 in]
